vi "Sensor Tests.vi"() -> ()   [LabVIEW 2012]
uses:
  Globals/Potentiometers.vi
  Globals/Encoders Global.vi
panel:
  out "Rate":dbl
  out "Act. Pot":dbl
  out "RR Pot":dbl
  out "RL Pot":dbl
  out "FR Pot":dbl
  out "FL Pot":dbl
  out "Shooter Codes":dbl
  out "RR Enc":dbl
  out "RL Enc":dbl
  out "FR Enc":dbl
  out "FL Enc":dbl
  out "IR":bool
  # "SWITCHBOX"
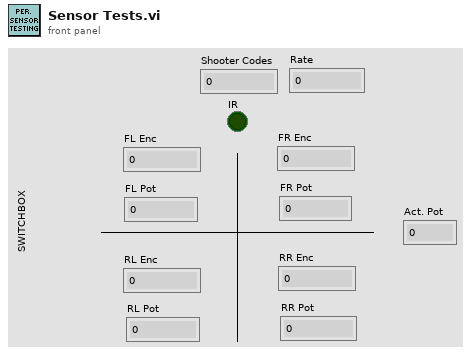
[diagram p1: front panel]
types:
  T1 = typedef "WPI_AnalogChannelDevRef.ctl" = cluster{"DevStatus":errorcluster, "Analog Module":T2, "Analog Channel":T3}
  T2 = typedef "FPGA_TypedefAnalogModule.ctl" = enum16{"Analog Module 1", "Analog Module 2"}
  T3 = typedef "FPGA_AIChannel.ctl" = enum8{"AI 1", "AI 2", "AI 3", "AI 4", "AI 5", "AI 6", "AI 7", "AI 8", "Invalid"}
  T4 = cluster{"Front Left":T1, "Front Right":T1, "Rear Left":T1, "Rear Right":T1, "Actuator":T1}
  T5 = typedef "WPI_EncoderDevRef.ctl" = cluster{"DevStatus":errorcluster, "EncoderIndex":T6, "CounterIndex":T7, "DistancePerCount":dbl, "Decoding Type":T8}
  T6 = typedef "FPGA_EncoderIdx.ctl" = enum8{"Enc 0", "Enc 1", "Enc 2", "Enc 3", "Invalid"}
  T7 = typedef "FPGA_CounterCtrSystemIndex.ctl" = enum8{"Ctr 0", "Ctr 1", "Ctr 2", "Ctr 3", "Ctr 4", "Ctr 5", "Ctr 6", "Ctr 7", "Invalid"}
  T8 = typedef "WPI_EncoderType.ctl" = enum16{"1x", "2x", "4x"}
  T9 = cluster{"Front Left":T5, "Front Right":T5, "Rear Left":T5, "Rear Right":T5, "Shooter":T5}
  T10 = typedef "WPI_DigitalInputDevRef.ctl" = cluster{"DevStatus":errorcluster, "DIO Channel":T11, "Digital Module":T12}
  T11 = typedef "FPGA_DIOChannel.ctl" = enum8{"DIO 1", "DIO 2", "DIO 3", "DIO 4", "DIO 5", "DIO 6", "DIO 7", "DIO 8", "DIO 9", "DIO 10", "DIO 11", "DIO 12", "DIO 13", "DIO 14", "Invalid"}
  T12 = typedef "FPGA_TypedefDigitalModule.ctl" = enum16{"Digital Module 1", "Digital Module 2"}
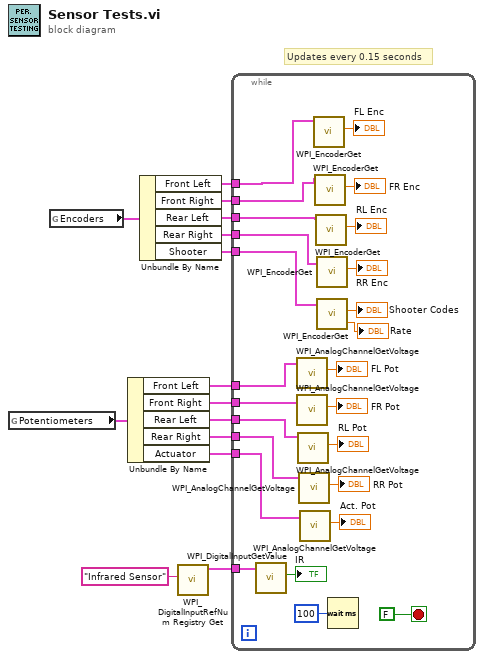
[diagram p0: block diagram]
diagram:
  # "Updates every 0.15 seconds"
  n1 = global read "Potentiometers.vi" "Potentiometers"() -> (w12:T4)
  n2 = global read "Encoders Global.vi" "Encoders"() -> (w6:T9)
  n3 = Unbundle By Name(w12) -> ("Front Left"=w11:T1, "Front Right"=w10:T1, "Rear Left"=w9:T1, "Rear Right"=w8:T1, "Actuator"=w7:T1)
  n4 = Unbundle By Name(w6) -> ("Front Left"=w5:T5, "Front Right"=w4:T5, "Rear Left"=w3:T5, "Rear Right"=w2:T5, "Shooter"=w1:T5)
  n5 = call <vilib>:"WPI_DigitalInputRefNum Registry Get.vi"("refnum name"="Infrared Sensor") -> ("DigitalInputDevRef"=w13:T10)  [unwired: 9 in, 1 out]
  n6 = while {
    tunnel: w13 -> [w25]
    tunnel: w11 -> [w24]
    tunnel: w10 -> [w23]
    tunnel: w9 -> [w22]
    tunnel: w8 -> [w21]
    tunnel: w7 -> [w20]
    tunnel: w5 -> [w19]
    tunnel: w4 -> [w18]
    tunnel: w3 -> [w17]
    tunnel: w2 -> [w16]
    tunnel: w1 -> [w15]
    stop <- FALSE stop-if-true
    n7 = call <vilib>:"WPI_DigitalInputGetValue.vi"("DigitalInputDevRef"=w25) -> ("Value"=→"IR":bool)  [unwired: 8 in, 2 out]
    n8 = call <vilib>:"WPI_AnalogChannelGetVoltage.vi"("AIDeviceRef"=w24) -> ("Voltage"=→"FL Pot":dbl)  [unwired: 8 in, 2 out]
    n9 = call <vilib>:"WPI_AnalogChannelGetVoltage.vi"("AIDeviceRef"=w23) -> ("Voltage"=→"FR Pot":dbl)  [unwired: 8 in, 2 out]
    n10 = call <vilib>:"WPI_AnalogChannelGetVoltage.vi"("AIDeviceRef"=w22) -> ("Voltage"=→"RL Pot":dbl)  [unwired: 8 in, 2 out]
    n11 = call <vilib>:"WPI_AnalogChannelGetVoltage.vi"("AIDeviceRef"=w21) -> ("Voltage"=→"RR Pot":dbl)  [unwired: 8 in, 2 out]
    n12 = call <vilib>:"WPI_AnalogChannelGetVoltage.vi"("AIDeviceRef"=w20) -> ("Voltage"=→"Act. Pot":dbl)  [unwired: 8 in, 2 out]
    n13 = call <vilib>:"WPI_EncoderGet.vi"("EncoderDevRef"=w19) -> ("Distance"=→"FL Enc":dbl)  [unwired: 5 in, 5 out]
    n14 = call <vilib>:"WPI_EncoderGet.vi"("EncoderDevRef"=w18) -> ("Distance"=→"FR Enc":dbl)  [unwired: 5 in, 5 out]
    n15 = call <vilib>:"WPI_EncoderGet.vi"("EncoderDevRef"=w17) -> ("Distance"=→"RL Enc":dbl)  [unwired: 5 in, 5 out]
    n16 = call <vilib>:"WPI_EncoderGet.vi"("EncoderDevRef"=w16) -> ("Distance"=→"RR Enc":dbl)  [unwired: 5 in, 5 out]
    n17 = call <vilib>:"WPI_EncoderGet.vi"("EncoderDevRef"=w15) -> ("Distance"=→"Shooter Codes":dbl, "Rate"=→"Rate":dbl)  [unwired: 5 in, 4 out]
    n18 = Wait (ms)(milliseconds to wait=u32 100) -> ()  [unwired: 1 out]
  }
